vi "sub_lane-pts_analysis.vi"(10 "clamp result out":T2 {"clamp_result"."ROI Descriptor out"."Contours"."Type" items=["No Selection", "Point", "Line", "Rectangle", "Oval", "Polygon", "Freehand Region", "Annulus", "Unused2", "Unused3", "Broken Line", "Freehand Line", "Rotated Rectangle"]}, 11 "lane points_in":cluster{"X":sgl, "Y":sgl}[](array[cluster])) -> (2 "analysis-result-b":bool[](array[boolean]), 3 "analysis-result":T3)   [LabVIEW 2019]
uses:
  Global_val.vi
  <vilib>/Analysis/NI_AALPro.lvlib
  <vilib>/Analysis/NI_AALBase.lvlib
panel:
  out "웨이브폼 차트 4":dbl(graph)
  out "웨이브폼 차트 3":cluster{"slope":dbl, "slope":dbl}(graph)
  out "웨이브폼 차트 2":dbl(graph)
  out "웨이브폼 차트":dbl(graph)
  out "웨이브폼 그래프":dbl[](graph)
  out "slope-l-b":bool
  out "slope-r-b":bool
  out "mean-y":dbl caption="mean_y" format="%0.2f"
  out "mean-x-c":dbl caption="mean_x" format="%0.2f"
  out "intercept-r":dbl
  out "intercept-l":dbl
  out "slope-r":dbl
  out "slope-l":dbl
  out "pts-r":i32
  out "pts-l":i32
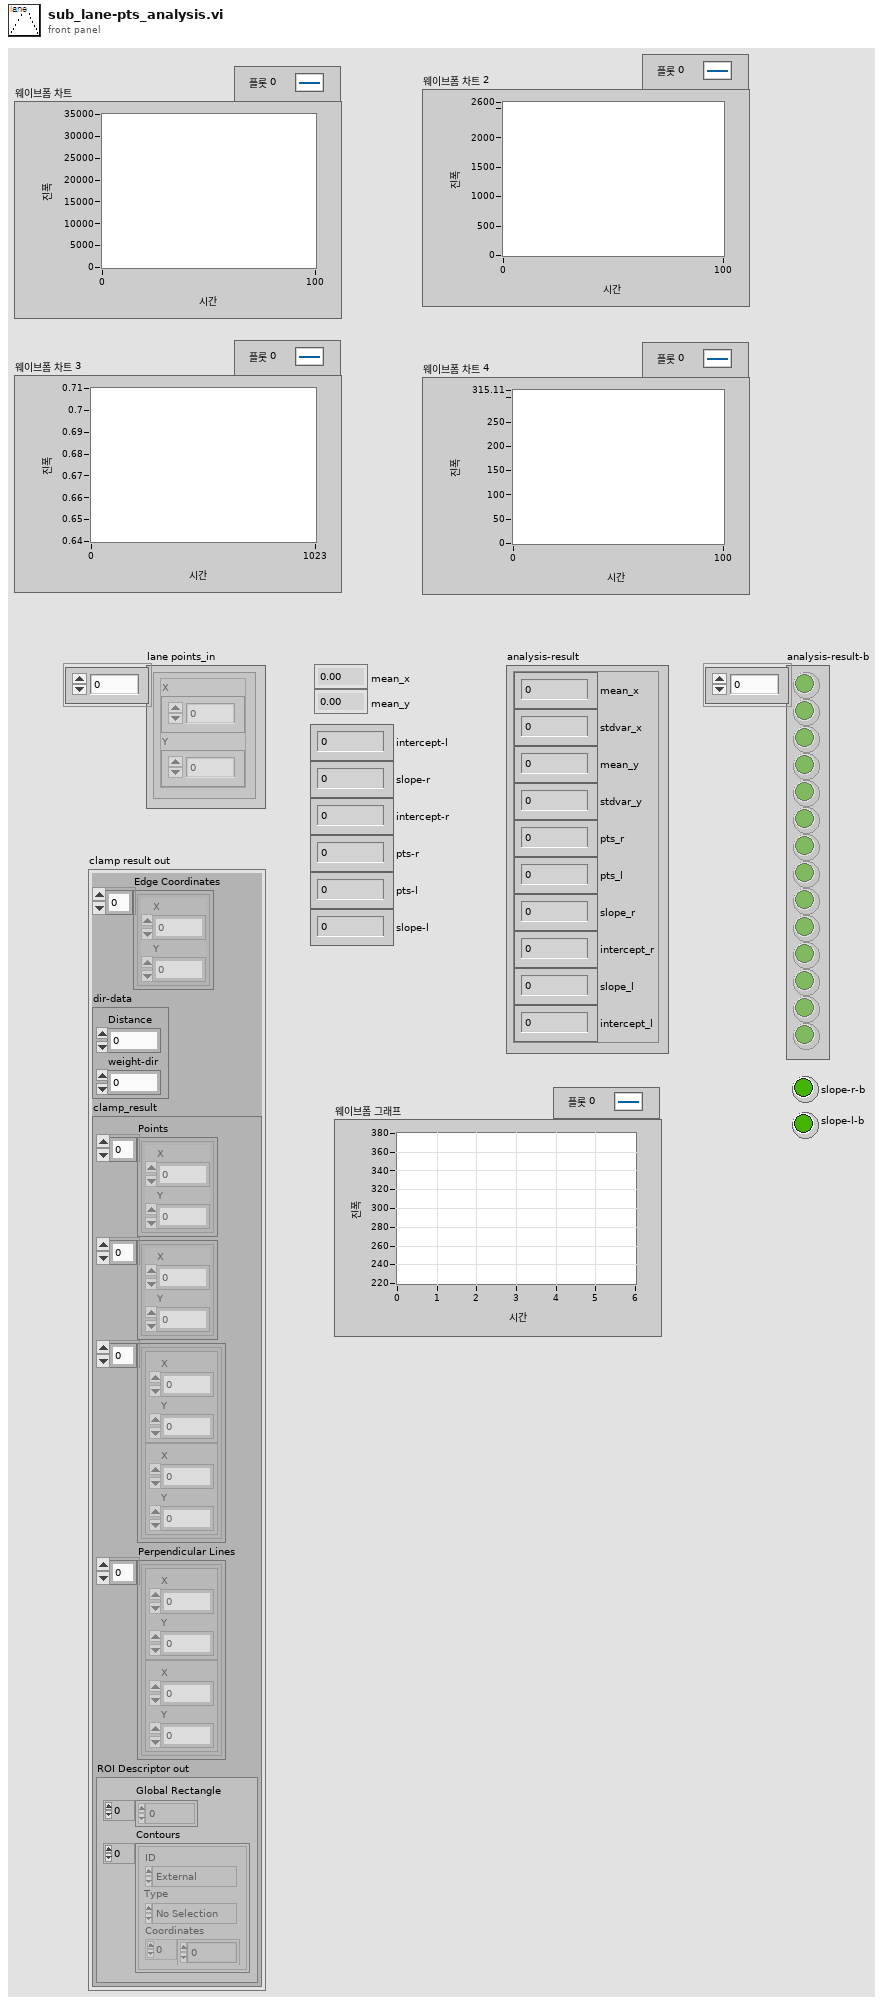
[diagram p1: front panel]
types:
  T1 = typedef "ROI Descriptor" = cluster{"Global Rectangle":i32[], "Contours":cluster{"ID":enum32{"External", "Internal"}, "Type":u32, "Coordinates":i32[]}[]}
  T2 = cluster{"Edge Coordinates":cluster{"X":sgl, "Y":sgl}[], "dir-data":cluster{"Distance":sgl, "weight-dir":dbl}, "clamp_result":cluster{"Points":cluster{"X":sgl, "Y":sgl}[], cluster{"X":sgl, "Y":sgl}[], cluster{cluster{"X":sgl, "Y":sgl}, cluster{"X":sgl, "Y":sgl}}[], "Perpendicular Lines":cluster{cluster{"X":sgl, "Y":sgl}, cluster{"X":sgl, "Y":sgl}}[], "ROI Descriptor out":T1}}
  T3 = cluster{"mean_x":dbl, "stdvar_x":dbl, "mean_y":dbl, "stdvar_y":dbl, "pts_r":i32, "pts_l":i32, "slope_r":dbl, "intercept_r":dbl, "slope_l":dbl, "intercept_l":dbl}
  T4 = cluster{"camera file path":path, "ROI-clamp":cluster{"Global Rectangle":i32[], "Contours":cluster{"Contour Type":u32, "ROI Type":u32, "Points":i32[]}[]}, "Clamp Settings":cluster{"Contrast":i32, "Filter width":i32, "Steepness":i32, "Subsampling Ratio":u32, "Show Search Area":bool, "Show Search Lines":bool, "Show Edges Found":bool, "Show Result":bool}, "Angle deg":sgl, "Image Size":cluster{"x":i32, "y":i32}, "x-center":dbl, "start_pt-l-out":i32[], "start_pt-r-out":i32[], "weight-ver-l":dbl, "weight-ver-r":dbl, "weight_hor":dbl, "Replace Value":sgl, "Threshold Range":cluster{"Lower value":sgl, "Upper value":sgl}, "video mode":u32}
  T5 = cluster{"mean":dbl, "variance":dbl, "mean":dbl, "variance":dbl, i32, i32, "slope":dbl, "intercept":dbl, "slope":dbl, "intercept":dbl}
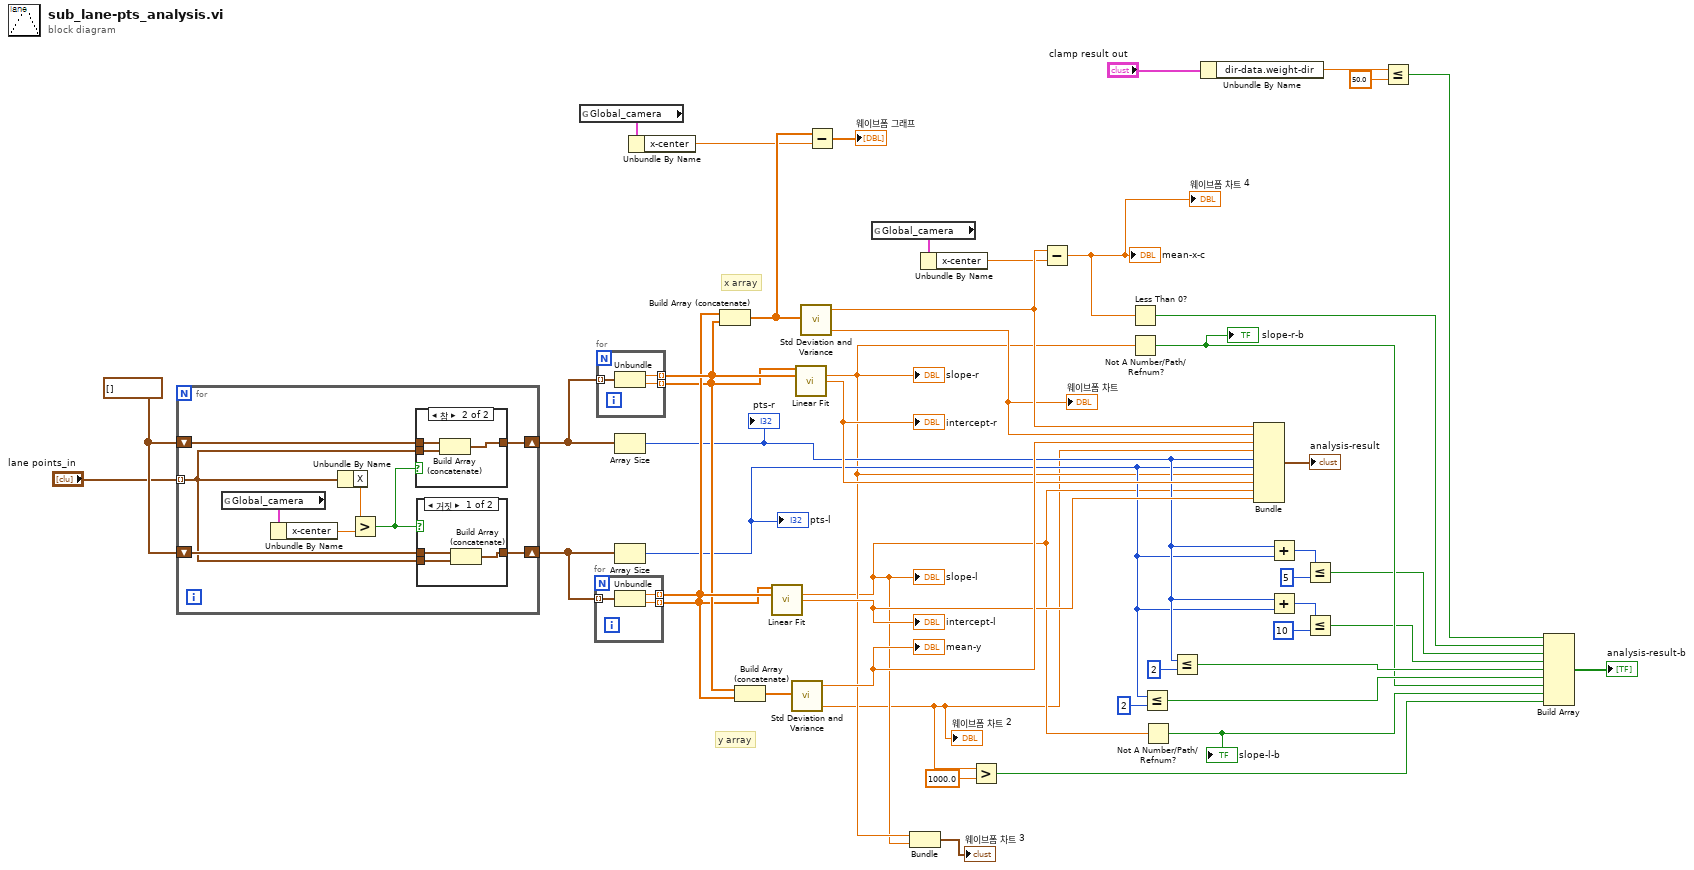
[diagram p0: block diagram]
diagram:
  w46 = cluster{"X":sgl, "Y":sgl}[] []
  # "y array"
  # "x array"
  n1 = for {
    tunnel: "lane points_in" -> [w51] mode=indexing
    shift-right: [w57] -> w47
    shift-left: w46 -> [w53]
    shift-right: [w55] -> w48
    shift-left: w46 -> [w56]
    n2 = global read "Global_val.vi" "Global_camera"() -> (w50:T4)
    n3 = Unbundle By Name(w50) -> ("x-center"=w49:dbl)
    n4 = Unbundle By Name(w51) -> ("X"=w54:sgl)
    n5 = Greater?(x=w54, y=w49) -> (0:w52:bool)
    n6 = case shown="참" w52 {
      tunnel: [w62 w65] -> w57
      tunnel: w51 -> [_ w64]
      tunnel: w53 -> [w62 w63]
      frame False {
      }
      frame True {
        n7 = Build Array (concatenate)(w63, w64) -> (w65:cluster{"X":sgl, "Y":sgl}[])
      }
    }
    n8 = case shown="거짓" w52 {
      tunnel: w56 -> [w60 w61]
      tunnel: [w59 w61] -> w55
      tunnel: w51 -> [w58 _]
      frame False {
        n9 = Build Array (concatenate)(w60, w58) -> (w59:cluster{"X":sgl, "Y":sgl}[])
      }
      frame True {
      }
    }
  }
  n10 = global read "Global_val.vi" "Global_camera"() -> (w22:T4)
  n11 = for {
    tunnel: w48 -> [w68] mode=indexing
    tunnel: [w67] -> w43 mode=indexing
    tunnel: [w66] -> w40 mode=indexing
    n12 = Unbundle(w68) -> ("X"=w67:sgl, "Y"=w66:sgl)
  }
  n13 = for {
    tunnel: w47 -> [w71] mode=indexing
    tunnel: [w70] -> w44 mode=indexing
    tunnel: [w69] -> w41 mode=indexing
    n14 = Unbundle(w71) -> ("X"=w70:sgl, "Y"=w69:sgl)
  }
  n15 = Array Size(array=w47) -> (size(s)=w12:i32)
  "pts-r" <- w12
  n16 = Array Size(array=w48) -> (size(s)=w11:i32)
  "pts-l" <- w11
  n17 = Unbundle By Name(w22) -> ("x-center"=w20:dbl)
  n18 = Build Array (concatenate)(w43, w44) -> (w21:sgl[])
  n19 = Build Array (concatenate)(w41, w40) -> (w42:sgl[])
  n20 = call <vilib>:"Linear Fit.vi"("Y"=w40, "X"=w43) -> ("slope"=w6:dbl, "intercept"=w37:dbl)  [unwired: 9 in, 3 out]
  "slope-l" <- w6
  "intercept-l" <- w37
  n21 = call <vilib>:"Std Deviation and Variance.vi"("X"=w42) -> ("mean"=w39:dbl, "variance"=w4:dbl)  [unwired: 1 in, 1 out]
  "mean-y" <- w39
  "웨이브폼 차트 2" <- w4
  n22 = call <vilib>:"Linear Fit.vi"("Y"=w41, "X"=w44) -> ("slope"=w7:dbl, "intercept"=w38:dbl)  [unwired: 9 in, 3 out]
  "slope-r" <- w7
  "intercept-r" <- w38
  n23 = call <vilib>:"Std Deviation and Variance.vi"("X"=w21) -> ("mean"=w24:dbl, "variance"=w9:dbl)  [unwired: 1 in, 1 out]
  "웨이브폼 차트" <- w9
  n24 = Subtract(x=w21, y=w20) -> (x-y=→"웨이브폼 그래프":dbl[])
  n25 = global read "Global_val.vi" "Global_camera"() -> (w25:T4)
  n26 = Bundle("slope"=w7, "slope"=w6) -> (→"웨이브폼 차트 3":cluster{"slope":dbl, "slope":dbl})  [unwired: 1 in]
  n27 = Unbundle By Name(w25) -> ("x-center"=w23:dbl)
  n28 = Greater?(x=w4, y=1000.0) -> (0:w1:bool)
  n29 = Subtract(x=w24, y=w23) -> (x-y=w8:dbl)
  "mean-x-c" <- w8
  "웨이브폼 차트 4" <- w8
  n30 = Less Than 0?(x=w8) -> (x < 0?=w15:bool)
  n31 = Not A Number/Path/Refnum?(number/path/refnum=w7) -> (NaN/Path/Refnum?=w26:bool)
  "slope-r-b" <- w26
  n32 = Less Or Equal?(x=w11, y=2) -> (x <= y?=w32:bool)
  n33 = Not A Number/Path/Refnum?(number/path/refnum=w6) -> (NaN/Path/Refnum?=w2:bool)
  "slope-l-b" <- w2
  n34 = Less Or Equal?(x=w12, y=2) -> (x <= y?=w33:bool)
  n35 = Unbundle By Name("clamp result out") -> ("dir-data.weight-dir"=w29:dbl)
  n36 = Bundle("mean"=w24, "variance"=w9, "mean"=w39, "variance"=w4, w12, w11, "slope"=w7, "intercept"=w38, "slope"=w6, "intercept"=w37) -> (→"analysis-result":T5)  [unwired: 1 in]
  n37 = Add(x=w12, y=w11) -> (x+y=w18:i32)
  n38 = Add(x=w12, y=w11) -> (x+y=w13:i32)
  n39 = Less Or Equal?(x=w18, y=5) -> (x <= y?=w16:bool)
  n40 = Less Or Equal?(x=w13, y=10) -> (x <= y?=w10:bool)
  n41 = Less Or Equal?(x=w29, y=50.0) -> (x <= y?=w27:bool)
  n42 = Build Array(w27, w15, w16, w10, w33, w32, w26, w2, w1) -> (→"analysis-result-b":bool[])
